vi "Bundle.vi"(8 "Aquirer Indices":i32[](array[numeric]), 9 "Aquirer":T1[](array[typedef]), 10 "Enqueue Locks":T2[](array[typedef]), 11 "Msg":refnum<class "Multi Instrument Msg.lvclass">) -> (3 "Multi Instrument Wrapper Msg out":refnum<class "Multi Instrument Wrapper Msg.lvclass">)   [LabVIEW 2020, in "Instrument Handler.lvlib" / "Multi Instrument Wrapper Msg.lvclass"]
doc: "Populate the Msg private data."
uses:
  Multi Instrument Wrapper Msg.lvclass
  Multi Instrument Msg/Multi Instrument Msg.lvclass
  Controls/Ctl_AquirerRefnum.ctl
  Multi Instrument Wrapper Msg.lvclass/Multi Instrument Wrapper Msg.ctl
  Instrument Handler.lvlib
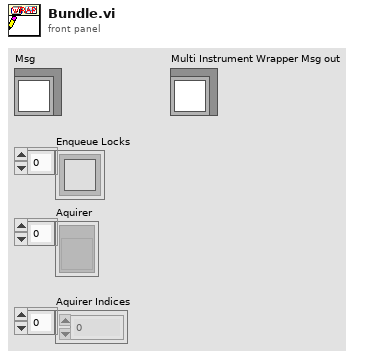
[diagram p1: front panel]
types:
  T1 = typedef "Instrument Handler.lvlib/Ctl_AquirerRefnum.ctl" = refnum<vi>
  T2 = typedef "Semaphore RefNum" = refnum<k1>
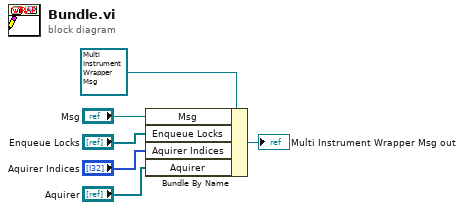
[diagram p0: block diagram]
diagram:
  n1 = Bundle By Name(cluster=refnum<class "Multi Instrument Wrapper Msg.lvclass"> refnum ("Multi Instrument Wrapper Msg in"), "Msg"="Msg", "Enqueue Locks"="Enqueue Locks", "Aquirer Indices"="Aquirer Indices", "Aquirer"="Aquirer") -> (→"Multi Instrument Wrapper Msg out":refnum<class "Multi Instrument Wrapper Msg.lvclass">)
